vi "CalcPeakArea.vi"(8 "spectrum":dbl[](array[numeric]), 9 "m/z in":dbl[](array[numeric]), 10 "to":dbl[](array[numeric]), 11 "from":dbl[](array[numeric])) -> (3 "Peak Area":dbl[](array[numeric]))   [LabVIEW 2012]
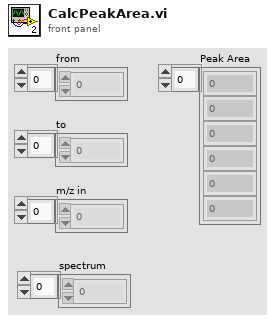
[diagram p1: front panel]
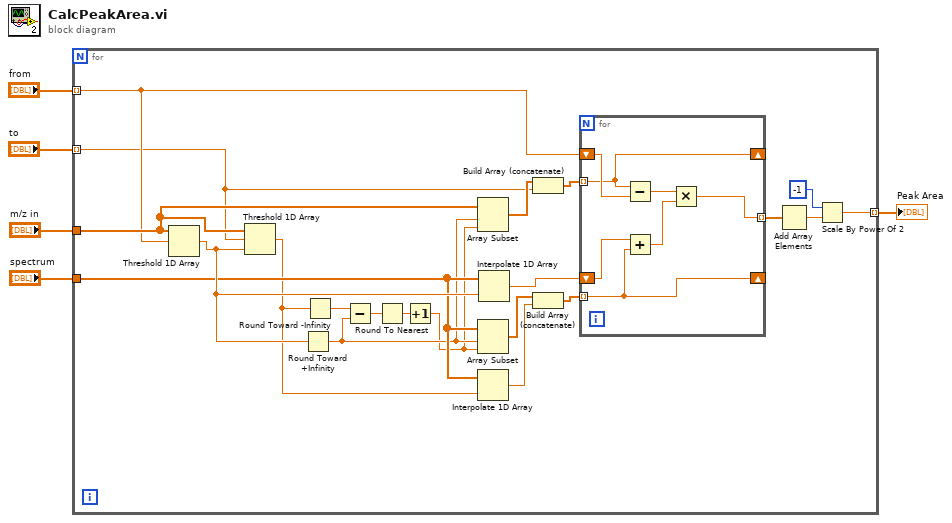
[diagram p0: block diagram]
diagram:
  n1 = for {
    tunnel: "m/z in" -> [w17]
    tunnel: "from" -> [w12] mode=indexing
    tunnel: "to" -> [w11] mode=indexing
    tunnel: [w7] -> w5 mode=indexing
    tunnel: "spectrum" -> [w23]
    n2 = Threshold 1D Array(2:w12, 3:w17) -> (0:w26:dbl)  [unwired: 1 in]
    n3 = Threshold 1D Array(1:w26, 2:w11, 3:w17) -> (0:w21:dbl)
    n4 = Round Toward +Infinity(x=w26) -> (ceil(x): smallest int >= x=w16:dbl)
    n5 = Round Toward -Infinity(1:w21) -> (0:w22:dbl)
    n6 = Subtract(x=w22, y=w16) -> (x-y=w25:dbl)
    n7 = Round To Nearest(number=w25) -> (nearest integer value=w24:dbl)
    n8 = Increment(x=w24) -> (x+1=w15:dbl)
    n9 = Array Subset(array=w17, index=w16, length=w15) -> (w14:dbl[])
    n10 = Array Subset(array=w23, index=w16, length=w15) -> (w20:dbl[])
    n11 = Interpolate 1D Array(1:w21, 2:w23) -> (0:w19:dbl)
    n12 = Interpolate 1D Array(1:w26, 2:w23) -> (0:w10:dbl)
    n13 = Build Array (concatenate)(w14, w11) -> (w13:dbl[])
    n14 = Build Array (concatenate)(w20, w19) -> (w18:dbl[])
    n15 = for {
      tunnel: w18 -> [w29] mode=indexing
      tunnel: w13 -> [w32] mode=indexing
      shift-right: [w32] -> _
      shift-left: w12 -> [w33]
      shift-right: [w29] -> _
      shift-left: w10 -> [w30]
      tunnel: [w27] -> w9 mode=indexing
      n16 = Subtract(x=w32, y=w33) -> (x-y=w31:dbl)
      n17 = Add(x=w30, y=w29) -> (x+y=w28:dbl)
      n18 = Multiply(x=w31, y=w28) -> (x*y=w27:dbl)
    }
    n19 = Add Array Elements(numeric array=w9) -> (sum=w8:dbl)
    n20 = Scale By Power Of 2(n=i16 -1, x=w8) -> (x*2^n=w7:dbl)
  }
  "Peak Area" <- w5
